vi "OpenAppRef.vi"(8 "error in (no error)":errorcluster, 9 "LVClass library Path":path, 11 "class reference":refnum<vi>) -> (0 "error out":errorcluster, 2 "Application reference":refnum<vi>, 3 "LVClass Reference":refnum<vi>)   [LabVIEW 2019, in "BlueUtilityScripts.lvlib"]
uses:
  BlueUtilityScripts.lvlib
  <vilib>/Utility/error.llb/Error Cluster From Error Code.vi
  <vilib>/ErrorRing/Error Ring.xnode
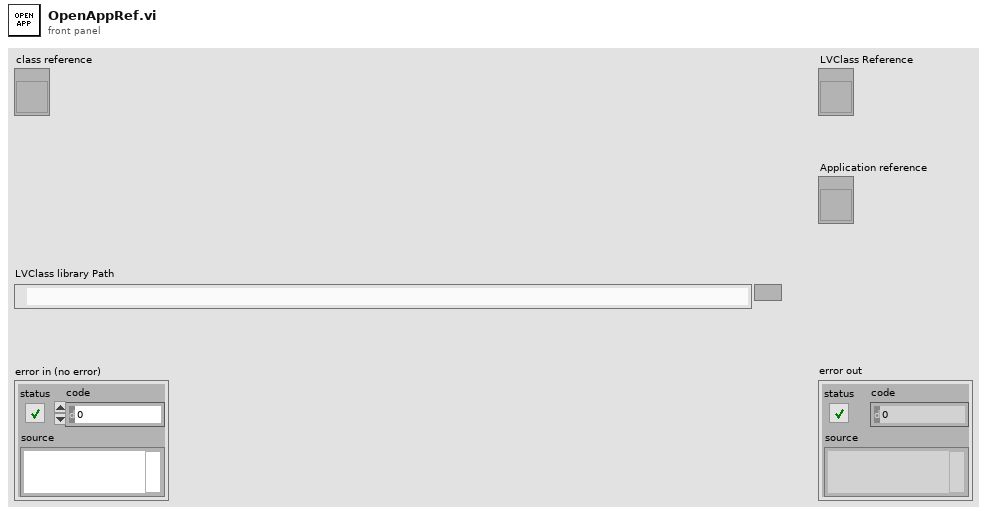
[diagram p1: front panel]
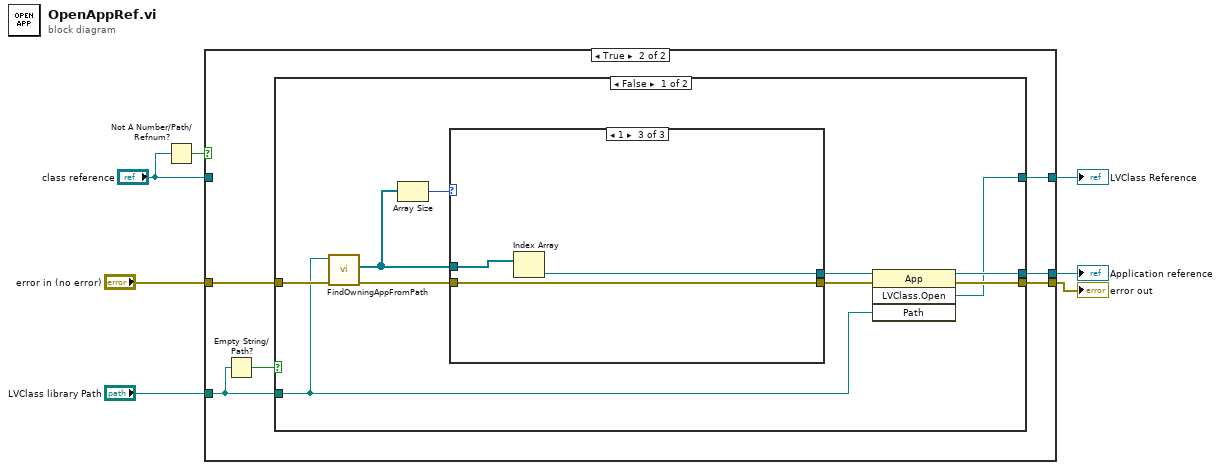
[diagram p0: block diagram]
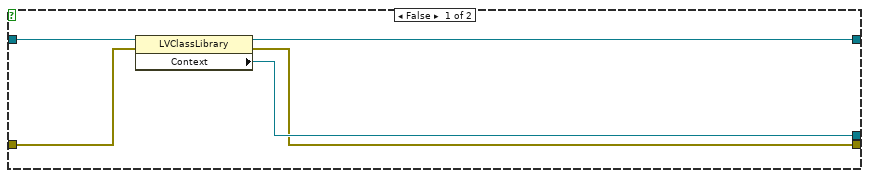
[diagram p2: hidden frame]
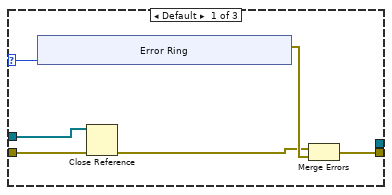
[diagram p3: hidden frame]
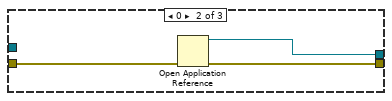
[diagram p4: hidden frame]
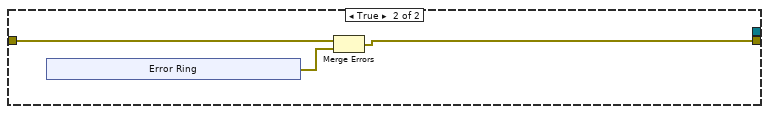
[diagram p5: hidden frame]
diagram:
  n1 = Not A Number/Path/Refnum?(number/path/refnum="class reference") -> (NaN/Path/Refnum?=w7:bool)
  n2 = case shown="True" w7 {
    tunnel: "class reference" -> [w12 _]
    tunnel: "LVClass library Path" -> [_ w14]
    tunnel: [w11 w17] -> w4
    tunnel: [w10 w15] -> w2
    tunnel: "error in (no error)" -> [w9 w18]
    tunnel: [w8 w16] -> w1
    frame False {
      n3 = property class="LVClassLibrary"(reference=w12, error in=w9) -> (reference out=w10:refnum<vi>, error out=w8:errorcluster, "Context"=w11:refnum<vi>)
    }
    frame True {
      n4 = Empty String/Path?(string/path=w14) -> (empty?=w13:bool)
      n5 = case shown="False" w13 {
        tunnel: w18 -> [w28 w49]
        tunnel: [w22 _] -> w17
        tunnel: [w21 w48] -> w16
        tunnel: [w20 _] -> w15
        tunnel: w14 -> [w19 _]
        frame False {
          n6 = call "FindOwningAppFromPath.vi"("error in (no error)"=w28, "LVClass path"=w19) -> ("error out"=w25:errorcluster, "owning applications"=w26:refnum<vi>[])  [unwired: 7 in, 1 out]
          n7 = Array Size(array=w26) -> (size(s)=w27:i32)
          n8 = case shown="1" w27 {
            selector: w27 -> [w34 _ _]
            tunnel: w26 -> [w31 _ w47]
            tunnel: [_ w44 w46] -> w24
            tunnel: w25 -> [w30 w43 w45]
            tunnel: [w32 w42 w45] -> w23
            frame Default {
              n9 = xnode "Error Ring"("parameter 0"=w34) -> ("error out"=w33:errorcluster)
              n10 = Close Reference(reference=w31, error in (no error)=w30) -> (error out=w29:errorcluster)
              n11 = Merge Errors(w29, w33) -> (w32:errorcluster)
            }
            frame 0 {
              n12 = Open Application Reference(8:w43) -> (0:w42:errorcluster, 3:w44:refnum<vi>)  [unwired: 3 in]
            }
            frame 1 {
              n13 = Index Array(array=w47) -> (element=w46:refnum<vi>)  [unwired: 1 in]
            }
          }
          n14 = invoke class="App" method="LVClass.Open"(reference=w24, error in=w23, "Path"=w19) -> (reference out=w22:refnum<vi>, error out=w21:errorcluster, "LVClass.Open"=w20:refnum<vi>)  [unwired: 1 in, 1 out]
        }
        frame True {
          n15 = xnode "Error Ring"() -> ("error out"=w50:errorcluster)
          n16 = Merge Errors(w49, w50) -> (w48:errorcluster)
        }
      }
    }
  }
  "Application reference" <- w4
  "error out" <- w1
  "LVClass Reference" <- w2
